vi "FPGA_recall-goto-values.vi"(11 "panel":u8 max=10 step=1) -> (1 "bus' goto values":u16[](array[numeric]))   [LabVIEW 2013]
uses:
  <vilib>/rvi/Memory/Memory_Emulation/nirvimemoryEmulation.vi
  <vilib>/rvi/Memory/Memory_Emulation/nirvimemoryFastEmulation.vi
  <vilib>/rvi/DataTransferAndStorage/Container/Common/niFpgaContainerGetUniqueNameForEmu.vi
  <vilib>/rvi/Memory/Memory_Emulation/niFpgaMemoryEmulationCacheClearOnFirstRun.vi
  <vilib>/rvi/Memory/Memory_Emulation/nirvimemoryEmulationManagerCache_MakeExclusive.vi
  <vilib>/rvi/Memory/Memory_Emulation/niFpgaMemoryEmulationValidateCache.vi
  <vilib>/rvi/Memory/Memory_Emulation/nirvimemoryEmulationManagerCache_ReleaseExclusive.vi
  <vilib>/rvi/Memory/Memory_Emulation/nirvimemoryEmulationManagerCache_InsertValue.vi
  <vilib>/Utility/error.llb/Clear Errors.vi
  <vilib>/rvi/Memory/Memory_Emulation/nirvimemoryEmulationManagerCache_GetValue.vi
  <vilib>/rvi/DataTransferAndStorage/Container/XNode/niFpgaContainer.xnode
panel:
  # "used to get goto values for a panel\nfrom memory and set them in an array"
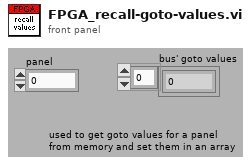
[diagram p1: front panel]
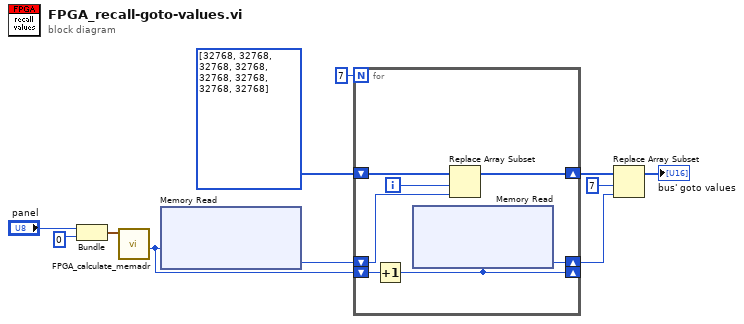
[diagram p0: block diagram]
diagram:
  n1 = Bundle("panel"="panel", u8 0) -> (w6:cluster{"panel":u8, u8})  [unwired: 1 out]
  n2 = call "FPGA_calculate_memadr.vi"("Cluster"=w6) -> ("mem adr"=w2:u8)  [unwired: 10 out]
  n3 = xnode ("Memory Read")("Address"=w2) -> ("Data"=w10:u16)  [unwired: 1 in, 1 out]
  n4 = for {
    N: 7 -> [_]
    shift-right: [w14] -> w8
    shift-left: w10 -> [w18]
    shift-right: [w16] -> w4
    shift-left: u16[] [32768, 32768, 32768, 32768, 32768, 32768, 32768, 32768] ("channels to") -> [w15]
    shift-right: [w12] -> _
    shift-left: w2 -> [w13]
    i -> [w17]
    n5 = Increment(x=w13) -> (x+1=w12:u8)
    n6 = xnode ("Memory Read")("Address"=w12) -> ("Data"=w14:u16)  [unwired: 1 in, 1 out]
    n7 = Replace Array Subset(array=w15, new element=w18, index=w17) -> (w16:u16[])
  }
  n8 = Replace Array Subset(array=w4, new element=w8, index=7) -> (→"bus' goto values":u16[])
